vi "Write Single Holding Register.vi"(8 "error in (no error)":errorcluster, 9 "holding register value":u16, 10 "address":u16, 11 "Modbus slave in":refnum<class "Modbus Slave.lvclass">) -> (0 "error out":errorcluster, 3 "Modbus slave out":refnum<class "Modbus Slave.lvclass">)   [LabVIEW 2021, in "Modbus Slave.lvclass"]
doc: "Writes a value to a single holding register."
uses:
  Modbus Slave.lvclass
  Modbus Slave.lvclass/Modbus Slave.ctl
  Data Model/Device Data Model.lvclass
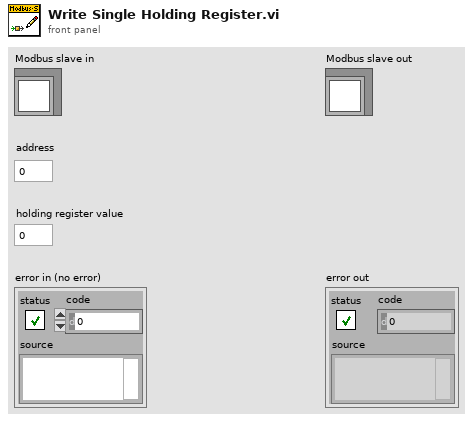
[diagram p1: front panel]
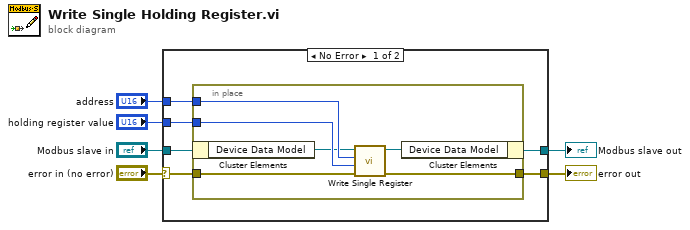
[diagram p0: block diagram]
diagram:
  n1 = case shown="No Error" "error in (no error)" {
    selector: "error in (no error)" -> [w9 w20]
    tunnel: [w12 w20] -> w3
    tunnel: "Modbus slave in" -> [w8 w19]
    tunnel: "holding register value" -> [w11 _]
    tunnel: "address" -> [w10 _]
    tunnel: [w7 w19] -> w1
    frame No Error {
      n2 = in-place {
        in-place-border: [w18] -> w12
        in-place-border: w11 -> [w17]
        in-place-border: w10 -> [w16]
        in-place-border: w9 -> [w15]
        n3 = in-place-cluster #1(w8) -> ("Device Data Model"=w14:refnum<class "Device Data Model.lvclass">)
        n4 = call-dynamic "Write Single Register.vi"("error in"=w15, "register value"=w17, "address"=w16, "device data model in"=w14) -> ("error out"=w18:errorcluster, "device data model out"=w13:refnum<class "Device Data Model.lvclass">)  [unwired: 6 in]
        n5 = in-place-cluster #1("Device Data Model"=w13) -> (w7:refnum<class "Modbus Slave.lvclass">)
      }
    }
    frame Error {
    }
  }
  "error out" <- w3
  "Modbus slave out" <- w1
